vi "ORS_Phase_Compensation_Fringes.vi"(5 "xi":dbl[](array[numeric]) format="%_6g", 6 "Do Interp":bool, 7 "X":dbl[](array[numeric]) format="%_6g", 8 "DualBackground":i16[](array[numeric]), 9 "Samples per line":i32, 10 "n_lines":i32, 11 "Raw Data":i16[](array[numeric])) -> (2 "dispcoef":dbl, 3 "PhaseCompVector":cdb[](array[numeric]))   [LabVIEW 2024]
uses:
  <vilib>/gmath/NI_Gmath.lvlib
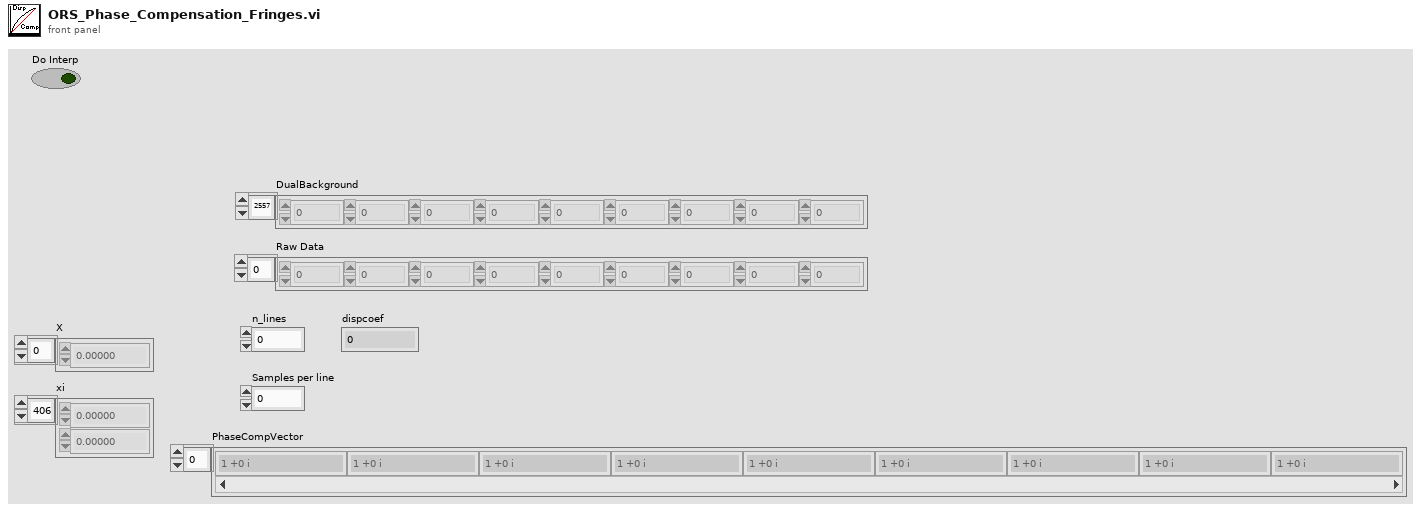
[diagram p1: front panel]
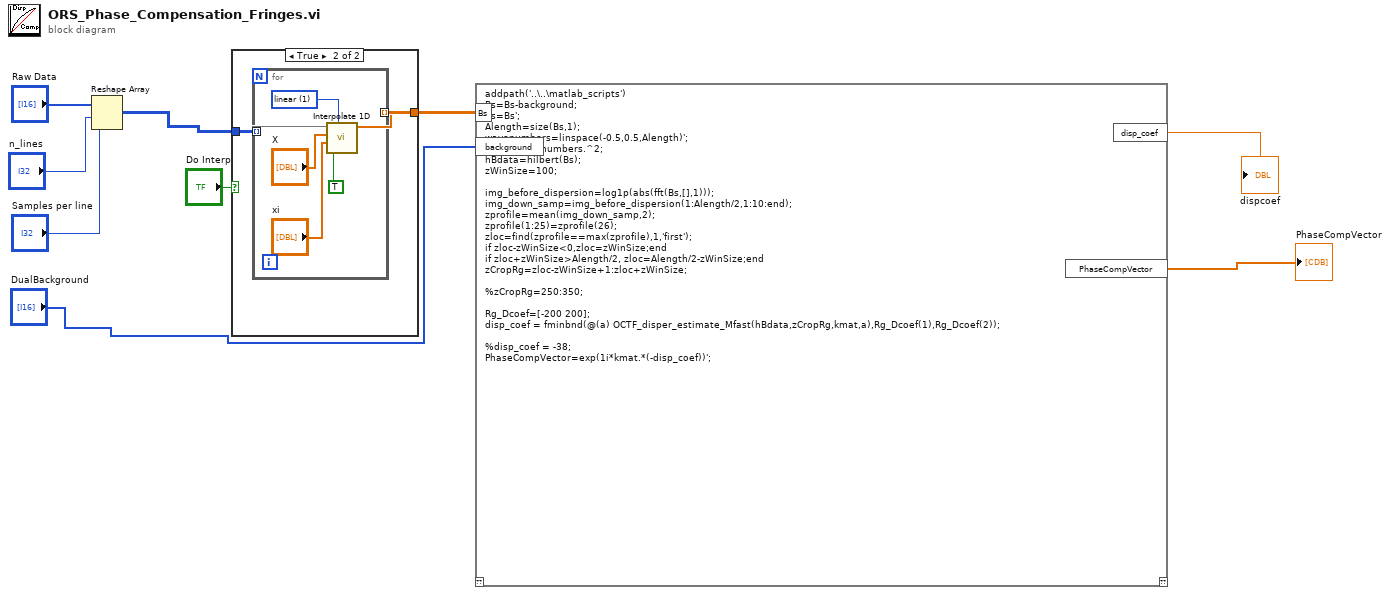
[diagram p0: block diagram]
diagram:
  n1 = Reshape Array("Raw Data", "n_lines", "Samples per line") -> (w2:i16[][])
  n2 = case shown="True" "Do Interp" {
    tunnel: w2 -> [w10 w12]
    tunnel: [w10 w11] -> w4
    frame False {
    }
    frame True {
      n3 = for {
        tunnel: w12 -> [w18] mode=indexing
        tunnel: [w17] -> w11 mode=indexing
        w14 = 1 items=["nearest", "linear", "spline", "cubic Hermite", "Lagrange"] ("method")
        n4 = call <vilib>:"Interpolate 1D.vi"("method"=w14, "X is monotonic"=TRUE, "xi"="xi", "X"="X", "Y"=w18) -> ("yi"=w17:dbl[])  [unwired: 4 in, 2 out]
      }
    }
  }
  n5 = script code="addpath('..\\..\\matlab_scripts')\nBs=Bs-background;\nBs=Bs';\nAlength=size(Bs,1);\nwavenumbers=linspace(-0.5,0.5,Alength)';\nkmat=wavenumbers.^2;\nhBdata=hilbert(Bs);\nzWinSize=100;\n\nimg_before_dispersion=log1p(abs(fft(Bs,[],1)));\nimg_down_samp=img_before_dispersion(1:Alength/2,1:10:end);\nzprofile=mean(img_down_samp,2);\nzprofile(1:25)=zprofile(26);\nzloc=find(zprofile==max(zprofile),1,'first');\nif zloc-zWinSize<0,zloc=zWinSize;end\nif zloc+zWinSize>Alength/2, zloc=Alength/2-zWinSize;end\nzCropRg=zloc-zWinSize+1:zloc+zWinSize;\n\n%zCropRg=250:350;\n\nRg_Dcoef=[-200 200];\ndisp_coef = fminbnd(@(a) OCTF_disper_estimate_Mfast(hBdata,zCropRg,kmat,a),Rg_Dcoef(1),Rg_Dcoef(2));\n\n%disp_coef = -38;\nPhaseCompVector=exp(1i*kmat.*(-disp_coef))';" ("Script Node")("Bs"=w4, "background"="DualBackground") -> ("PhaseCompVector"=→"PhaseCompVector":cdb[], "disp_coef"=→"dispcoef":dbl)  [unwired: 1 in, 1 out]
